vi "Update Water Level.vi"(8 "error in (no error)":cluster{"状态":bool, "代码":i32, "源":string} caption="错误输入（无错误）", 10 "水位":dbl, 11 "冷却器UI输入":refnum<class "Live User Controller.lvclass">) -> (0 "error out":cluster{"状态":bool, "代码":i32, "源":string} caption="错误输出", 3 "冷却器UI输出":refnum<class "Live User Controller.lvclass">)   [LabVIEW 2015, in "Live User Controller.lvclass"]
doc: "更新用户接口，显示水位。"
uses:
  Live User Controller.lvclass
  Live User Controller.lvclass/Live User Controller.ctl
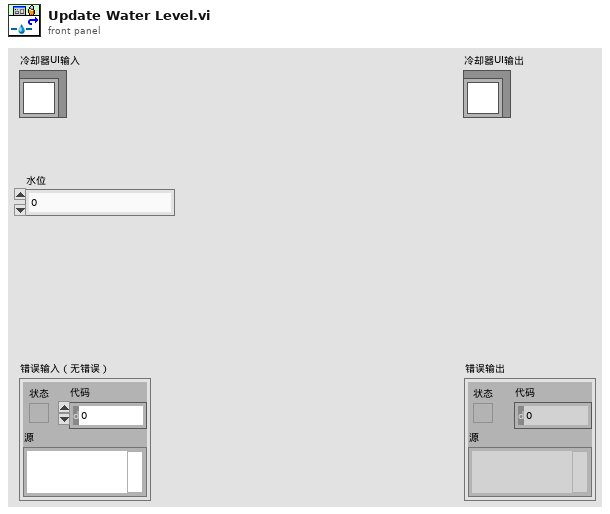
[diagram p1: front panel]
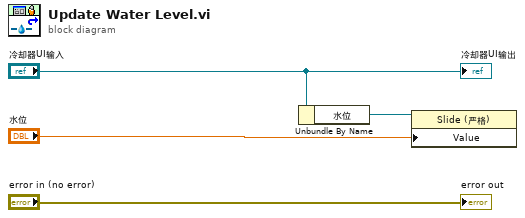
[diagram p0: block diagram]
diagram:
  n1 = Unbundle By Name("冷却器UI输入") -> ("水位"=w1:refnum<vi>)
  n2 = property class="Slide (严格)"(reference=w1, "Value"="水位") -> ()  [unwired: 1 in, 2 out]
  "error out" <- "error in (no error)"
  "冷却器UI输出" <- "冷却器UI输入"
